vi "DIAdem Param CSB.vi"(4 "error in (no error)":errorcluster, 6 "Parameter":string, 7 "File Directory":path) -> (0 "error out":errorcluster, 3 "DIAdem Command Parameter":string)   [LabVIEW 2017]
doc: "This VI bundles special additional DIAdem start parameters."
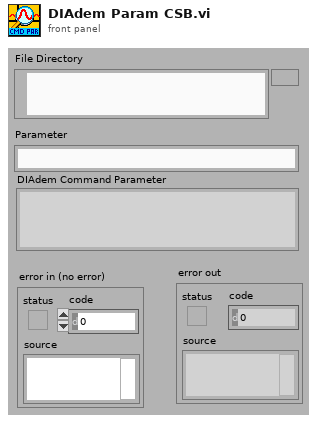
[diagram p1: front panel]
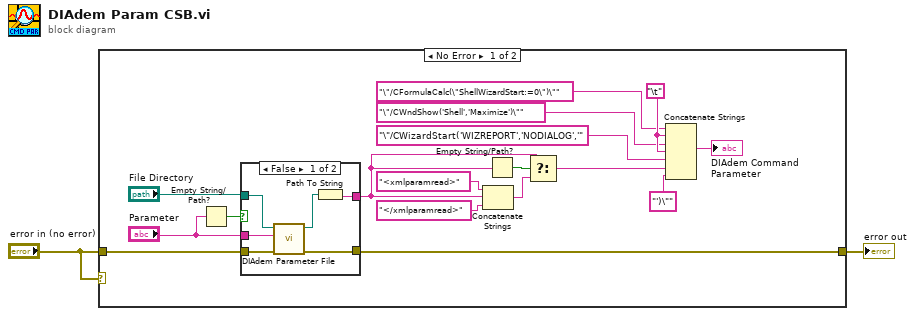
[diagram p0: block diagram]
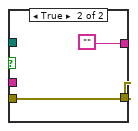
[diagram p2: hidden frame]
diagram:
  n1 = case shown="No Error" "error in (no error)" {
    tunnel: "error in (no error)" -> [w14 w28]
    tunnel: [w13 w28] -> w1
    frame No Error {
      w5 = "\t"
      n2 = Empty String/Path?(string/path="Parameter") -> (empty?=w11:bool)
      n3 = case shown="False" w11 {
        tunnel: w14 -> [w25 w27]
        tunnel: [w24 w27] -> w13
        tunnel: "File Directory" -> [w23 _]
        tunnel: "Parameter" -> [w22 _]
        tunnel: [w20 ""] -> w9
        frame False {
          n4 = call <vilib>:"DIAdem Parameter File.vi"("error in (no error)"=w25, "Parameter"=w22, "File Directory"=w23) -> ("error out"=w24:errorcluster, "Parameter File"=w21:path)  [unwired: 3 in]
          n5 = Path To String(path=w21) -> (string=w20:string)
        }
        frame True {
        }
      }
      n6 = Concatenate Strings("<xmlparamread>", w9, "</xmlparamread>") -> (w18:string)
      n7 = Empty String/Path?(string/path=w9) -> (empty?=w17:bool)
      n8 = Select(t=w9, s=w17, f=w18) -> (s? t:f=w7:string)
      n9 = Concatenate Strings("\"/CFormulaCalc(\"ShellWizardStart:=0\")\"" ("DIAdem Command"), w5, "\"/CWndShow('Shell','Maximize')\"", w5, "\"/CWizardStart('WIZREPORT','NODIALOG','" ("command"), w7, "')\"" ("Substring")) -> (→"DIAdem Command Parameter":string)
    }
    frame Error {
    }
  }
  "error out" <- w1
